vi "Kinesis-program-two-motor-Old-Controllers.vi"() -> ()   [LabVIEW 2014]
doc: "André Romero - 2017\nandretec@ifsc.usp.br"
uses:
  C:/user-Lab/AndreTec/GITs/andretec/Thorlabs-Vector-Move/kinesisTec/Kinesis/Thorlabs.MotionControl.Controls.dll
  kinesisTec/Kinesis/Thorlabs.MotionControl.Controls.dll
panel:
  out "GetPOS X 2":dbl=10.0 format="%^#1_6e"
  out "Refnum out 2":refnum<k24>
  out "Motor 2":bool
  out "Refnum out 1":refnum<k24>
  out "GetPOS X":dbl=10.0 format="%^#1_6e"
  in  "GO Move":bool
  out "Motor 1":bool
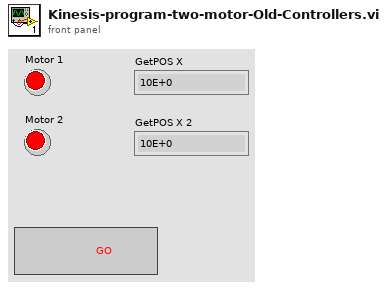
[diagram p1: front panel]
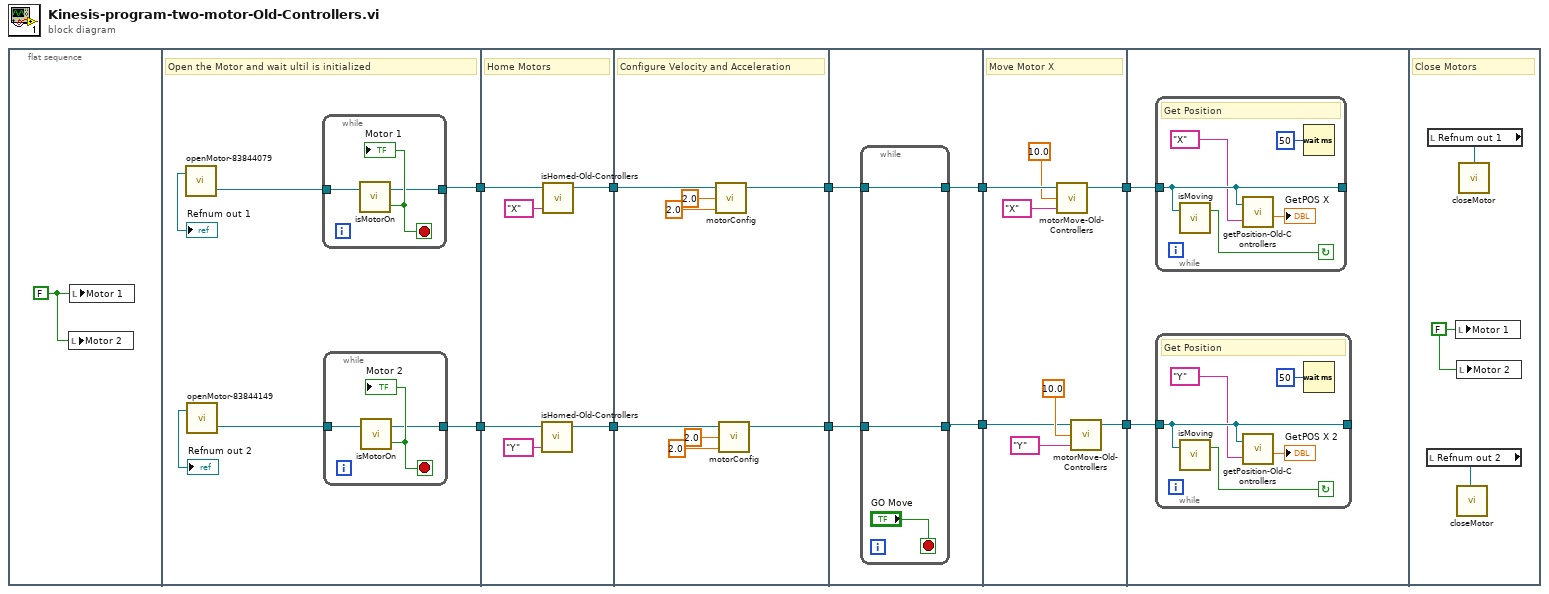
[diagram p0: block diagram]
diagram:
  n1 = flat-sequence {
    tunnel: [w17] -> w6
    tunnel: [w12] -> w5
    tunnel: w6 -> [w29]
    tunnel: [w28] -> w10
    tunnel: w5 -> [w25]
    tunnel: [w24] -> w4
    tunnel: w10 -> [w34]
    tunnel: [w35] -> w9
    tunnel: w4 -> [w31]
    tunnel: [w30] -> w3
    tunnel: w9 -> [w40]
    tunnel: [w41] -> w8
    tunnel: w3 -> [w39]
    tunnel: [w38] -> w2
    tunnel: w8 -> [w52]
    tunnel: [w51] -> w7
    tunnel: w2 -> [w46]
    tunnel: [w45] -> w1
    tunnel: w7 -> [w54]
    tunnel: w1 -> [w53]
    frame #0 {
      w11 = FALSE ("isConnected")
      n2 = local write "Motor 2"(w11) -> ()
      n3 = local write "Motor 1"(w11) -> ()
    }
    frame #1 {
      # "Open the Motor and wait ultil is initialized"
      n4 = call "openMotor-83844079.vi"() -> ("Device"=w16:refnum<k24>, ".NET Refnum out"=→"Refnum out 1":refnum<k24>)  [unwired: 2 in]
      n5 = call "openMotor-83844149.vi"() -> ("Device"=w14:refnum<k24>, ".NET Refnum out"=→"Refnum out 2":refnum<k24>)  [unwired: 2 in]
      n6 = while {
        tunnel: [w21] -> w17
        tunnel: w16 -> [w22]
        stop <- w23 stop-if-true
        n7 = call "isMotorOn.vi"("Device"=w22) -> ("isConnected"=w23:bool, "Device out"=w21:refnum<k24>)  [unwired: 1 in]
        "Motor 1" <- w23
      }
      n8 = while {
        tunnel: [w18] -> w12
        tunnel: w14 -> [w19]
        stop <- w20 stop-if-true
        n9 = call "isMotorOn.vi"("Device"=w19) -> ("isConnected"=w20:bool, "Device out"=w18:refnum<k24>)  [unwired: 1 in]
        "Motor 2" <- w20
      }
    }
    frame #2 {
      # "Home Motors"
      n10 = call "isHomed-Old-Controllers.vi"("Motor (XYZ)"="Y", "Device in"=w25) -> ("Device out"=w24:refnum<k24>)  [unwired: 3 in]
      n11 = call "isHomed-Old-Controllers.vi"("Motor (XYZ)"="X", "Device in"=w29) -> ("Device out"=w28:refnum<k24>)  [unwired: 3 in]
    }
    frame #3 {
      # "Configure Velocity and Acceleration"
      n12 = call "motorConfig.vi"("Velocity"=2.0 ("MaxVelocity"), "Acceleration"=2.0, "Device in"=w34) -> ("Device out"=w35:refnum<k24>)  [unwired: 2 in]
      n13 = call "motorConfig.vi"("Velocity"=2.0 ("MaxVelocity"), "Acceleration"=2.0, "Device in"=w31) -> ("Device out"=w30:refnum<k24>)  [unwired: 2 in]
    }
    frame #4 {
      n14 = while {
        tunnel: [w43] -> w41
        tunnel: w40 -> [w43]
        tunnel: w39 -> [w42]
        tunnel: [w42] -> w38
        stop <- "GO Move" stop-if-true
      }
    }
    frame #5 {
      # "Move Motor X"
      n15 = call "motorMove-Old-Controllers.vi"("Motor (XYZ)"="X", "position"=10.0, "Device in"=w52) -> ("Device out"=w51:refnum<k24>)  [unwired: 2 in]
      n16 = call "motorMove-Old-Controllers.vi"("Motor (XYZ)"="Y", "position"=10.0, "Device in"=w46) -> ("Device out"=w45:refnum<k24>)  [unwired: 2 in]
    }
    frame #6 {
      n17 = while {
        tunnel: w54 -> [w62]
        tunnel: [w62] -> _
        stop <- w64 continue-if-true
        # "Get Position"
        n18 = call "isMoving.vi"("Device in"=w62) -> ("IsMoving"=w64:bool)  [unwired: 1 in, 1 out]
        n19 = call "getPosition-Old-Controllers.vi"("Motor (XYZ)"="X", "Device"=w62) -> ("GetPOS"=→"GetPOS X":dbl)  [unwired: 1 in]
        n20 = Wait (ms)(milliseconds to wait=u32 50) -> ()  [unwired: 1 out]
      }
      n21 = while {
        tunnel: w53 -> [w57]
        tunnel: [w57] -> _
        stop <- w59 continue-if-true
        # "Get Position"
        n22 = call "isMoving.vi"("Device in"=w57) -> ("IsMoving"=w59:bool)  [unwired: 1 in, 1 out]
        n23 = call "getPosition-Old-Controllers.vi"("Motor (XYZ)"="Y", "Device"=w57) -> ("GetPOS"=→"GetPOS X 2":dbl)  [unwired: 1 in]
        n24 = Wait (ms)(milliseconds to wait=u32 50) -> ()  [unwired: 1 out]
      }
    }
    frame #7 {
      w65 = FALSE ("Motor 1")
      # "Close Motors"
      n25 = local read "Refnum out 2"() -> (w66:refnum<k24>)
      n26 = local read "Refnum out 1"() -> (w67:refnum<k24>)
      n27 = local write "Motor 1"(w65) -> ()
      n28 = local write "Motor 2"(w65) -> ()
      n29 = call "closeMotor.vi"(".NET Refnum in"=w66) -> ()  [unwired: 2 in]
      n30 = call "closeMotor.vi"(".NET Refnum in"=w67) -> ()  [unwired: 2 in]
    }
  }
